vi "PLC设备关闭.vi"(8 "error in (no error)":errorcluster caption="错误输入（无错误）", 11 "PLC设置":T1={"ActLogicalStationNumber"=9600, "ActUtlType"=refnum}) -> (0 "error out":errorcluster caption="错误输出", 2 "返回值":i32, 3 "PLC设置2":T1)   [LabVIEW 2015, in "Action.lvlib"]
uses:
  Action.lvlib
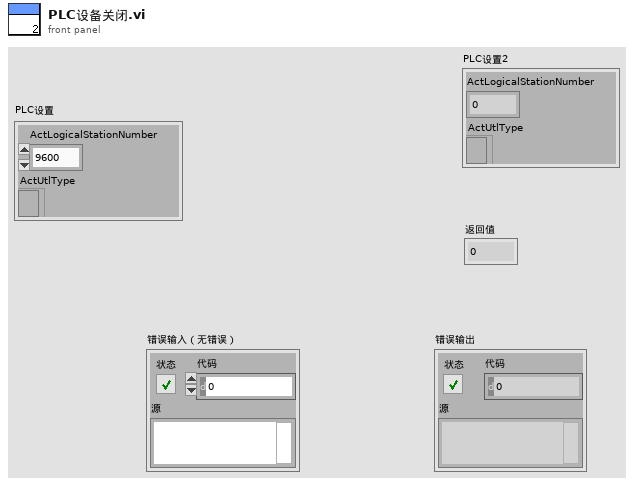
[diagram p1: front panel]
types:
  T1 = typedef "Action.lvlib/PLC设置.ctl" = cluster{"ActLogicalStationNumber":i32, "ActUtlType":refnum<k7>}
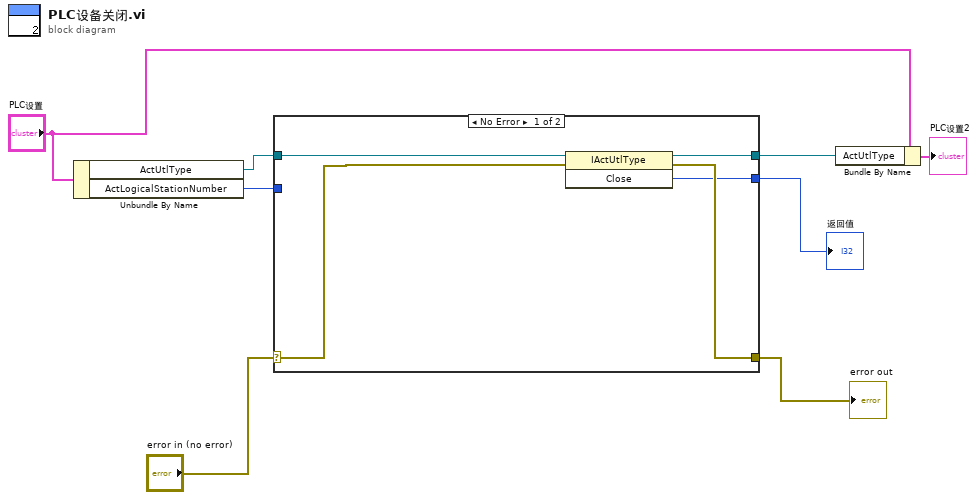
[diagram p0: block diagram]
diagram:
  n1 = Unbundle By Name("PLC设置") -> ("ActUtlType"=w4:refnum<k7>, "ActLogicalStationNumber"=w6:i32)
  n2 = case shown="No Error" "error in (no error)" {
    selector: "error in (no error)" -> [w10 w15]
    tunnel: [w13 w15] -> w7
    tunnel: w6 -> [_ _]
    tunnel: w4 -> [w9 w14]
    tunnel: [w12 _] -> w5
    tunnel: [w11 w14] -> w2
    frame No Error {
      n3 = invoke class="IActUtlType" method="Close"(reference=w9, error in=w10) -> (reference out=w11:refnum<k7>, error out=w13:errorcluster, "Close"=w12:i32)  [unwired: 1 in]
    }
    frame Error {
    }
  }
  "error out" <- w7
  "返回值" <- w5
  n4 = Bundle By Name(cluster="PLC设置", "ActUtlType"=w2) -> (→"PLC设置2":T1)
